vi "SinglePoint.vi"(8 "Error In 2":errorcluster, 11 "Async State Vars 2":T1) -> (0 "Error Out":errorcluster, 3 "Async State Vars out":T1)   [LabVIEW 2015, in "Waveform-Processing-Custom-Device Shared.lvlib" / "SinglePoint.lvlib"]
uses:
  SinglePoint.lvlib
  Engine/Types/AsyncStateVariables.ctl
  <vilib>/NI Veristand/Custom Device Waveform API/Single Waveform Read (DBL)/Single Waveform Read (DBL).lvclass
  <vilib>/NI Veristand/Custom Device Waveform API/Single Waveform Write (DBL)/Single Waveform Write (DBL).lvclass
  <vilib>/NI Veristand/Custom Device API/Waveform Data Reference.ctl
  <vilib>/ni/NIVS Inline Async API/_Data Access Engine/Data Access Engine/Types/Write.DVR.ctl
  <vilib>/ni/NIVS Inline Async API/_Data Access Engine/Access Type Classes/Write/Write.lvclass
  <vilib>/ni/NIVS Inline Async API/_Data Access Engine/Data Access Engine/Types/Read.DVR.ctl
  <vilib>/ni/NIVS Inline Async API/_Data Access Engine/Access Type Classes/Read/Read.lvclass
  <userlib>/Circular Buffer/Controls/Circular Buffer Operations.ctl
  <vilib>/ni/NIVS Inline Async API/_Data Access Engine/Access Type Classes/Write/Write.lvclass/Write.ctl
  <vilib>/ni/NIVS Inline Async API/_Data Access Engine/Data Access Engine/Methods/Write.Data.vi
  <vilib>/ni/NIVS Inline Async API/_Data Access Engine/Access Type Classes/Write/Write.ProcessData.vi
  <userlib>/Circular Buffer/Instance VIs/Circular Buffer(2D DBL).vi
  <userlib>/Circular Buffer/Circular Buffer.lvlib
  <vilib>/ni/NIVS Inline Async API/_Data Access Engine/Data Access Engine/Data Access Engine.lvclass
  <vilib>/NI VeriStand/Custom Device API/Custom Device API.lvlib
  Engine/Waveform-Processing-Custom-Device Engine.lvlib
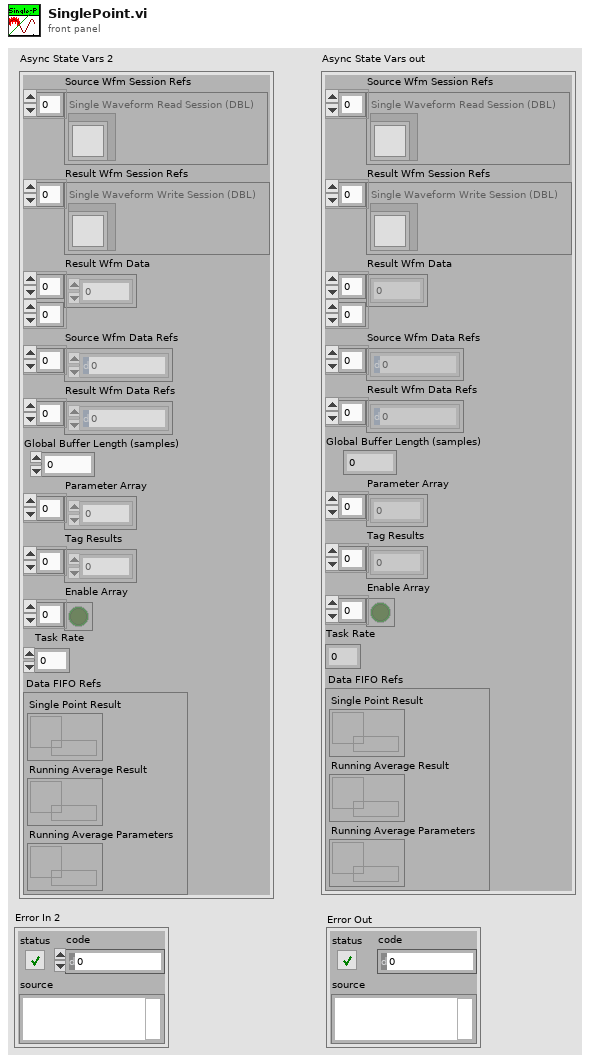
[diagram p1: front panel]
types:
  T1 = typedef "Waveform-Processing-Custom-Device Engine.lvlib/AsyncStateVariables.ctl" = cluster{"Source Wfm Session Refs":refnum<class "Single Waveform Read (DBL).lvclass">[], "Result Wfm Session Refs":refnum<class "Single Waveform Write (DBL).lvclass">[], "Result Wfm Data":dbl[][], "Source Wfm Data Refs":T2[], "Result Wfm Data Refs":T2[], "Global Buffer Length (samples)":dbl, "Parameter Array":dbl[], "Tag Results":dbl[], "Enable Array":bool[], "Task Rate":dbl, "Data FIFO Refs":cluster{"Single Point Result":T3, "Running Average Result":T3, "Running Average Parameters":T4}}
  T2 = typedef "Custom Device API.lvlib/Waveform Data Reference.ctl" = i32
  T3 = typedef "Data Access Engine.lvlib/Data Access Engine.lvclass/Write.DVR.ctl" = refnum<data-value>
  T4 = typedef "Data Access Engine.lvlib/Data Access Engine.lvclass/Read.DVR.ctl" = refnum<data-value>
  T5 = typedef "Circular Buffer.lvlib/Circular Buffer Operations.ctl" = enum16{"Initialize", "Get Backlog", "Write", "Read (continuous)", "Read (most recent)"}
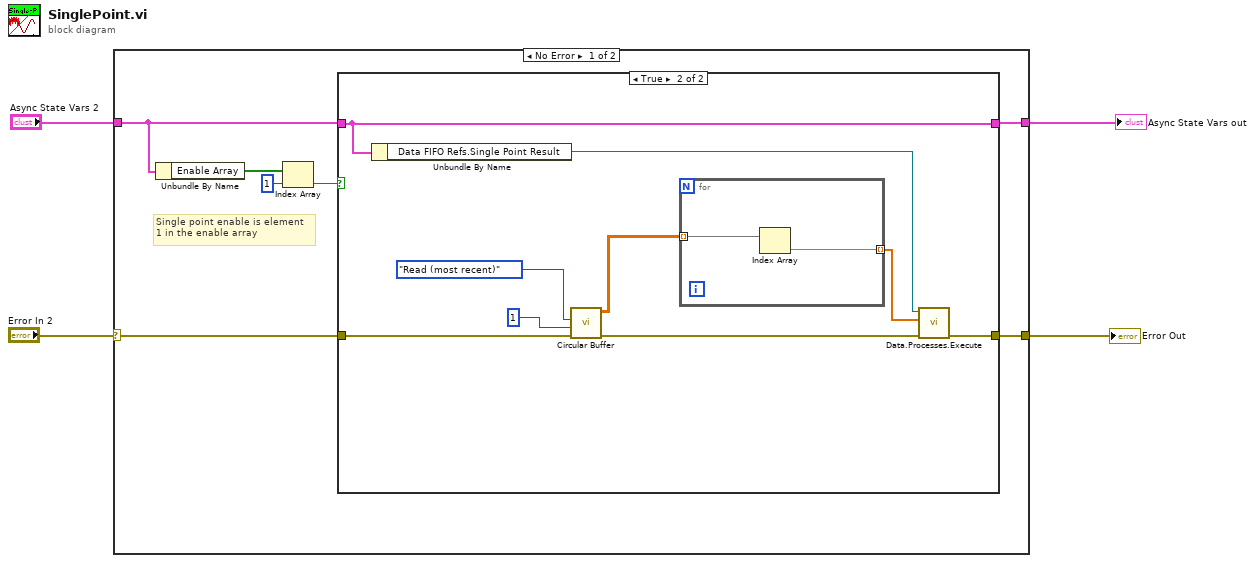
[diagram p0: block diagram]
diagram:
  n1 = case shown="No Error" "Error In 2" {
    selector: "Error In 2" -> [w11 w26]
    tunnel: [w10 w26] -> w2
    tunnel: "Async State Vars 2" -> [w8 w25]
    tunnel: [w9 w25] -> w4
    frame No Error {
      # "Single point enable is element\n1 in the enable array"
      n2 = Unbundle By Name(w8) -> ("Enable Array"=w7:bool[])
      n3 = Index Array(array=w7, index=1) -> (element=w5:bool)
      n4 = case shown="True" w5 {
        tunnel: w11 -> [w13 w21]
        tunnel: [w13 w17] -> w10
        tunnel: [w12 w19] -> w9
        tunnel: w8 -> [w12 w19]
        frame False {
        }
        frame True {
          n5 = Unbundle By Name(w19) -> ("Data FIFO Refs.Single Point Result"=w16:T3)
          n6 = call-poly <userlib>:"Circular Buffer.vi"("error in (no error)"=w21, "Read Size"=1, "Operation"=Circular_Buffer_Operations."Read (most recent)") -> ("error out"=w18:errorcluster, "Data Out"=w14:dbl[][])  [unwired: 5 in, 2 out]
          n7 = for {
            tunnel: w14 -> [w24] mode=indexing
            tunnel: [w23] -> w15 mode=indexing
            n8 = Index Array(array=w24) -> (element=w23:dbl)  [unwired: 1 in]
          }
          n9 = call-poly <vilib>:"Data.Processes.Execute.vi"("error in (no error)"=w18, "Values"=w15, "Ref"=w16) -> ("error out"=w17:errorcluster)  [unwired: 8 in]
        }
      }
    }
    frame Error {
    }
  }
  "Error Out" <- w2
  "Async State Vars out" <- w4
